vi "Get Wfm Names and Suggest New Name.vi"(8 "error in (no error)":errorcluster, 11 "Wfm Ref In":refnum<vi>) -> (0 "error out":errorcluster, 1 "New Wfm Name":string, 2 "Wfm Names":string[](array[string]), 3 "Wfm Ref Out":refnum<vi>)   [LabVIEW 2025, in "Fgen Script Mode UI.lvlib"]
uses:
  Fgen Script Mode UI.lvlib
  Typedef/Wfm Typedef.ctl
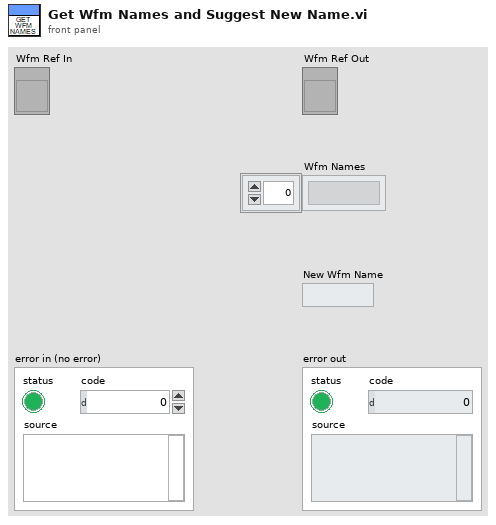
[diagram p1: front panel]
types:
  T1 = typedef "Fgen Script Mode UI.lvlib/Wfm Typedef.ctl" = cluster{"Name":string, "Path":string, "Grp":string, "Chn":string}
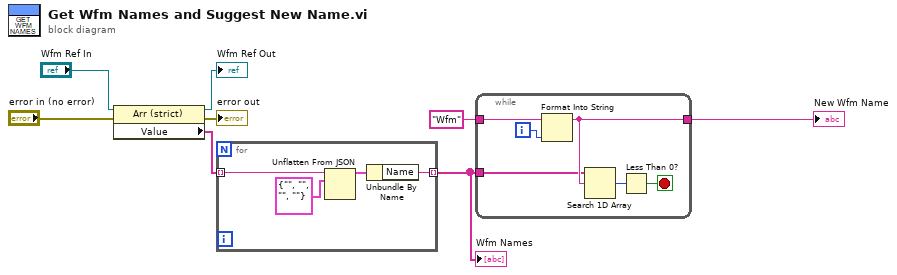
[diagram p0: block diagram]
diagram:
  n1 = property class="Arr (strict)"(reference="Wfm Ref In", error in="error in (no error)") -> (reference out=→"Wfm Ref Out":refnum<vi>, error out=→"error out":errorcluster, "Value"=w5:string[])
  n2 = for {
    tunnel: w5 -> [w11] mode=indexing
    tunnel: [w9] -> w6 mode=indexing
    n3 = Unflatten From JSON(JSON string=w11, type and defaults=T1 {"Name"="", "Path"="", "Grp"="", "Chn"=""} ("Waveform")) -> (value=w10:T1)  [unwired: 5 in, 1 out]
    n4 = Unbundle By Name(w10) -> ("Name"=w9:string)
  }
  "Wfm Names" <- w6
  n5 = while {
    tunnel: "Wfm" -> [w18]
    tunnel: [w14] -> w7
    tunnel: w6 -> [w13]
    i -> [w17]
    stop <- w15 stop-if-true
    n6 = Format Into String(initial string=w18, w17) -> (resulting string=w14:string)  [unwired: 2 in, 1 out]
    n7 = Search 1D Array(1D array=w13, element=w14) -> (index of element=w16:i32)  [unwired: 1 in]
    n8 = Less Than 0?(x=w16) -> (x < 0?=w15:bool)
  }
  "New Wfm Name" <- w7
